vi "Destroy View.vi"(0 "Abstract View in":refnum<class "Abstract View.lvclass">, 11 "error in (no error)":errorcluster) -> (4 "Abstract View out":refnum<class "Abstract View.lvclass">, 15 "error out":errorcluster)   [LabVIEW 2022 SP3, in "Abstract View.lvlib" / "Abstract View.lvclass"]
uses:
  Abstract View.lvclass
  Abstract View.lvclass/Abstract View.ctl
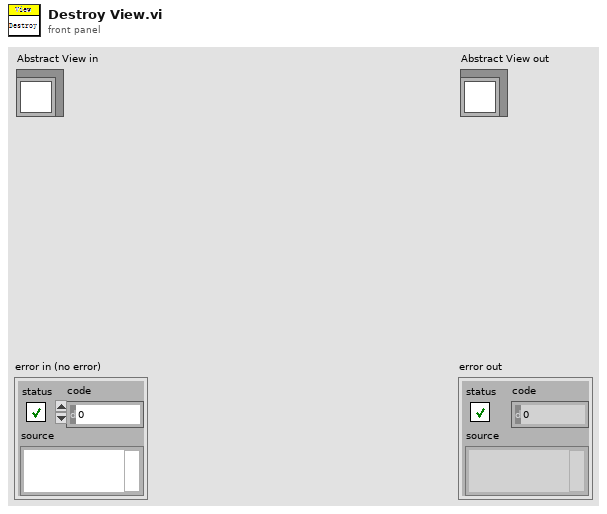
[diagram p1: front panel]
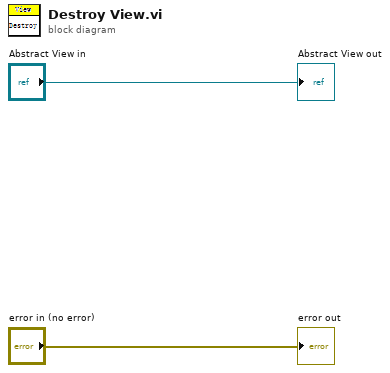
[diagram p0: block diagram]
diagram:
  "error out" <- "error in (no error)"
  "Abstract View out" <- "Abstract View in"
